vi "Send Software Trigger [SWT] Core.vi"(8 "error in (no error)":errorcluster, 11 "IVI_DCPwr in":refnum<class "IVI_DCPwr.lvclass">) -> (0 "error out":errorcluster, 3 "IVI_DCPwr out":refnum<class "IVI_DCPwr.lvclass">)   [LabVIEW 2016, in "IVI_DCPwr.lvlib" / "IVI_DCPwr.lvclass"]
doc: "This VI sends a command to trigger the power supply. Call this VI if you configure the power supply to respond to software triggers. If the power supply is not configured to respond to software triggers, this VI returns the error IVIDCPWR_ERROR_TRIGGER_NOT_SOFTWARE (0xBFFA1001).\n\nNotes:\n\n(1) This VI is part of the IviDCPwrSoftwareTrigger [SWT] extension group."
uses:
  IVI_DCPwr.lvclass
  IVI_DCPwr.lvclass/IVI_DCPwr.ctl
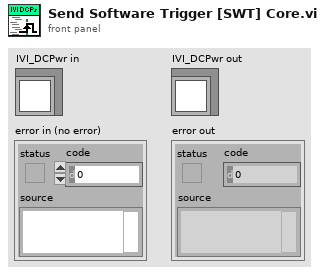
[diagram p1: front panel]
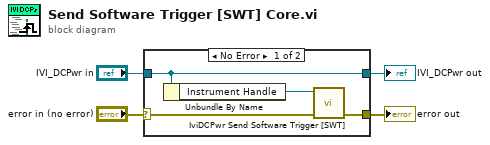
[diagram p0: block diagram]
diagram:
  n1 = case shown="No Error" "error in (no error)" {
    selector: "error in (no error)" -> [w6 w10]
    tunnel: [w5 w10] -> w3
    tunnel: [w8 w9] -> w1
    tunnel: "IVI_DCPwr in" -> [w8 w9]
    frame No Error {
      n2 = Unbundle By Name(w8) -> ("Instrument Handle"=w7:refnum<k15>)
      n3 = call <vilib>:"IviDCPwr Send Software Trigger [SWT].vi"("error in (no error)"=w6, "instrument handle"=w7) -> ("error out"=w5:errorcluster)  [unwired: 8 in, 1 out]
    }
    frame Error {
    }
  }
  "error out" <- w3
  "IVI_DCPwr out" <- w1
